vi "Time-Delayed Response.vi"(8 "error in (no error)":errorcluster, 11 "Timer in":refnum<class "Timer.lvclass">) -> (0 "error out":errorcluster, 3 "Timer out":refnum<class "Timer.lvclass">)   [LabVIEW 2016, in "Timer.lvclass"]
uses:
  Timer.lvclass
  C:/github/Measure_core/da Base/da Base.lvclass
  da Base/da Base.lvclass/da Base.ctl
  Timer.lvclass/Timer.ctl
  Results/Acquired Result/Acquired Result.lvclass
  <vilib>/express/express signal manip/GetorSetDDTAttributes/Shared VIs/TimeType.ctl
  Results/Acquired Result/Acquired Result.lvclass/Acquired Result.ctl
  Results/Acquired Result/Write Channels.vi
  Results/Acquired Result/Write Sender.vi
  Results/Acquired Result/Write Group.vi
  da Base/Read Active.vi
  da Base/Read Reply to.vi
  Read Latest time.vi
  da Base/Read Name.vi
  da Base/Write Active.vi
  <vilib>/express/express signal manip/GetorSetDDTAttributes/Shared VIs/TimeMode Enum to Boolean.vi
  <vilib>/express/express shared/transition.llb/Dynamic To Waveform Array.vi
  <vilib>/express/express signal manip/GetorSetDDTAttributes/Set DDT Attributes/SetT0.vi
  <vilib>/express/express shared/transition.llb/Waveform Array To Dynamic.vi
  Da Base Messages/Result Reply Msg/Result Reply Msg.lvclass
  <vilib>/express/express signal manip/GetorSetDDTAttributes/Set DDT Attributes/Set DDT Properties.xnode
  <vilib>/express/express signal manip/GetorSetDDTAttributes/Shared VIs/GetSetShared.lvlib
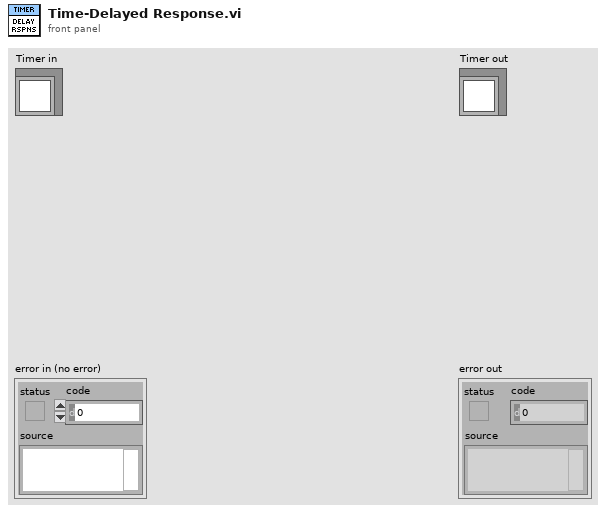
[diagram p1: front panel]
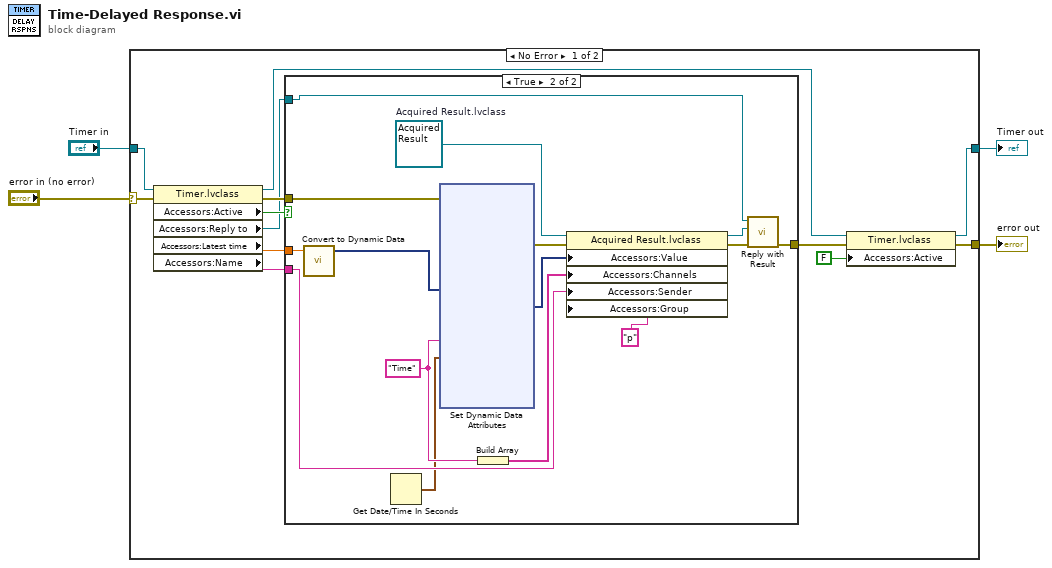
[diagram p0: block diagram]
diagram:
  n1 = case shown="No Error" "error in (no error)" {
    selector: "error in (no error)" -> [w9 w61]
    tunnel: [w5 w61] -> w3
    tunnel: [w8 w60] -> w1
    tunnel: "Timer in" -> [w16 w60]
    frame No Error {
      n2 = property class="Timer.lvclass"(reference=w16, error in=w9) -> (reference out=w15:refnum<class "Timer.lvclass">, error out=w12:errorcluster, "Accessors:Active"=w14:bool, "Accessors:Reply to"=w10:refnum<class "Result Reply Msg.lvclass">, "Accessors:Latest time"=w13:dbl, "Accessors:Name"=w11:string)
      n3 = case shown="True" w14 {
        tunnel: w13 -> [_ w26]
        tunnel: w12 -> [w17 w20]
        tunnel: w11 -> [_ w31]
        tunnel: w10 -> [_ w30]
        tunnel: [w17 w27] -> w7
        frame False {
        }
        frame True {
          w23 = "Time" ("String")
          w32 = refnum<class "Acquired Result.lvclass"> refnum  # Acquired Result.lvclass
          n4 = call "Convert to Dynamic Data"("Double"=w26) -> ("Dynamic Data Type"=w25:dynamicdata)  [unwired: 3 in]
          n5 = Get Date/Time In Seconds() -> (seconds since 1Jan1904=w22:timestamp)
          n6 = xnode "Set Dynamic Data Attributes"("Signals In"=w25, "Signal Name"=w23, "Timestamp"=w22, "error in"=w20) -> ("Signals Out"=w21:dynamicdata, "error out"=w19:errorcluster)  [unwired: 3 in]
          n7 = Build Array(w23) -> (w24:string[])
          n8 = property class="Acquired Result.lvclass"(reference=w32, error in=w19, "Accessors:Value"=w21, "Accessors:Channels"=w24, "Accessors:Sender"=w31, "Accessors:Group"="p" ("Group")) -> (reference out=w29:refnum<class "Acquired Result.lvclass">, error out=w28:errorcluster)
          n9 = call-dynamic "Reply with Result.vi"("error in (no error)"=w28, "Result"=w29, "Result Reply Msg in"=w30) -> ("error out"=w27:errorcluster)  [unwired: 7 in, 1 out]
        }
      }
      n10 = property class="Timer.lvclass"(reference=w15, error in=w7, "Accessors:Active"=FALSE) -> (reference out=w8:refnum<class "Timer.lvclass">, error out=w5:errorcluster)
    }
    frame Error {
    }
  }
  "error out" <- w3
  "Timer out" <- w1
